vi "ReleaseUTMgrRes.vi"(8 "错误输入（无错误）":errorcluster) -> (0 "错误输出":errorcluster)   [LabVIEW 2018]
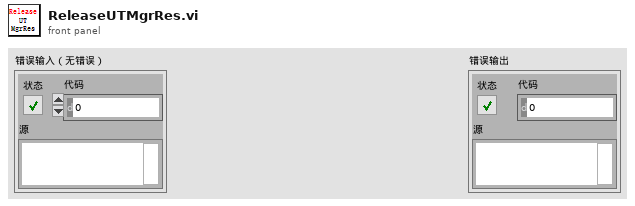
[diagram p1: front panel]
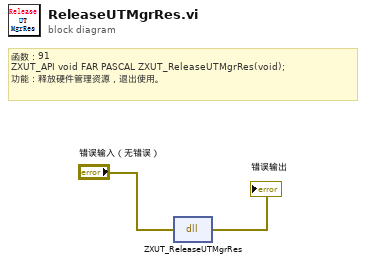
[diagram p0: block diagram]
diagram:
  # "函数：91\nZXUT_API void\tFAR PASCAL ZXUT_ReleaseUTMgrRes(void);\t\n功能：释放硬件管理资源，退出使用。"
  n1 = dll-call lib="PTH2Rabs E软件项目超声超声子VI函数VI\tTCG处理ZXUTConfigMgr.dll" fn="ZXUT_ReleaseUTMgrRes"(error in="错误输入（无错误）") -> (error out=→"错误输出":errorcluster)  [unwired: 3 in, 1 out]
